vi "LH6HDmessage_inycom.vi"(10 "DeviceAddress":u8, 11 "MessageType":T1(ring)) -> (3 "Message":string)   [LabVIEW 2015]
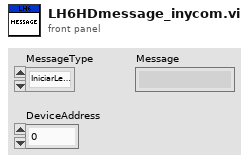
[diagram p1: front panel]
types:
  T1 = enum16{"IniciarLectura", "SolicitarEstado", "SolicitarTag", "Inhibir"}
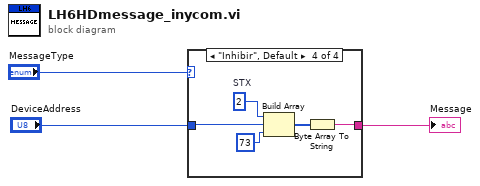
[diagram p0: block diagram]
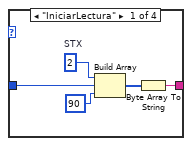
[diagram p2: hidden frame]
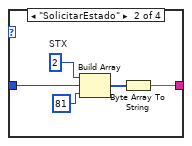
[diagram p3: hidden frame]
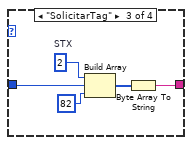
[diagram p4: hidden frame]
diagram:
  n1 = case shown="\"Inhibir\", Default" "MessageType" {
    tunnel: [w4 w10 w14 w19] -> w3
    tunnel: "DeviceAddress" -> [w5 w9 w15 w20]
    frame "IniciarLectura" {
      w6 = u8 2  # STX
      n2 = Build Array(w6, w5, u8 90 ("element")) -> (w7:u8[])
      n3 = Byte Array To String(unsigned byte array=w7) -> (string=w4:string)
    }
    frame "SolicitarEstado" {
      w11 = u8 2  # STX
      n4 = Build Array(w11, w9, u8 81 ("element")) -> (w12:u8[])
      n5 = Byte Array To String(unsigned byte array=w12) -> (string=w10:string)
    }
    frame "SolicitarTag" {
      w16 = u8 2  # STX
      n6 = Build Array(w16, w15, u8 82 ("element")) -> (w17:u8[])
      n7 = Byte Array To String(unsigned byte array=w17) -> (string=w14:string)
    }
    frame "Inhibir", Default {
      w21 = u8 2  # STX
      n8 = Build Array(w21, w20, u8 73 ("element")) -> (w22:u8[])
      n9 = Byte Array To String(unsigned byte array=w22) -> (string=w19:string)
    }
  }
  "Message" <- w3
